vi "XML array.vi"(8 "tag":string, 11 "String":string) -> (3 "Array":string[](array[string]))   [LabVIEW 2013]
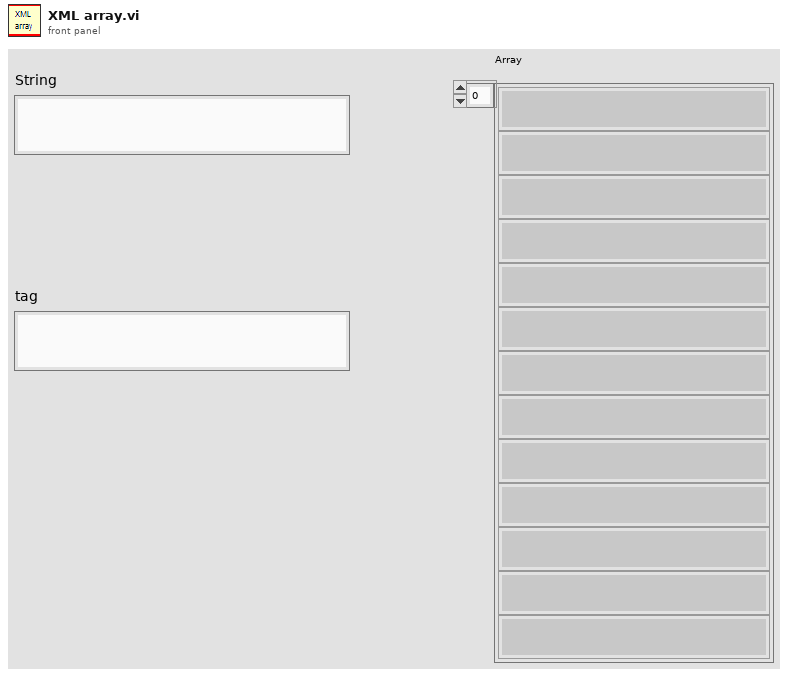
[diagram p1: front panel]
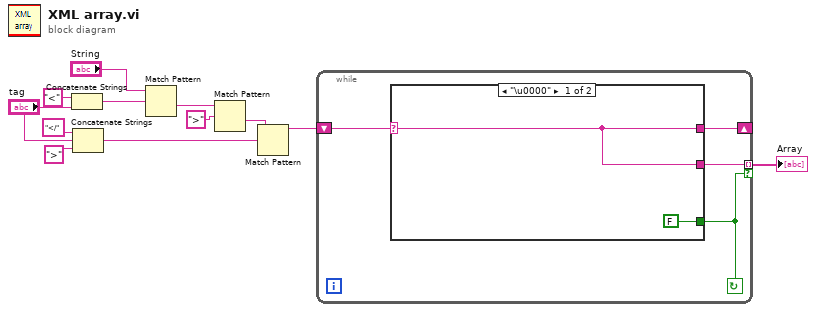
[diagram p0: block diagram]
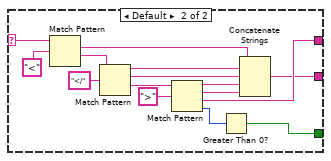
[diagram p2: hidden frame]
diagram:
  n1 = Concatenate Strings("<" ("string"), "tag") -> (w4:string)
  n2 = Concatenate Strings("</" ("string"), "tag", ">" ("string")) -> (w3:string)
  n3 = Match Pattern(string="String", regular expression=w4) -> (after substring=w11:string)  [unwired: 1 in, 3 out]
  n4 = Match Pattern(string=w11, regular expression=">") -> (after substring=w9:string)  [unwired: 1 in, 3 out]
  n5 = Match Pattern(string=w9, regular expression=w3) -> (before substring=w2:string)  [unwired: 1 in, 3 out]
  n6 = while {
    shift-right: [w16] -> _
    shift-left: w2 -> [w14]
    tunnel: [w15] -> w1 mode=indexing if=w13
    stop <- w13 continue-if-true
    n7 = case shown="\"\"" w14 {
      selector: w14 -> [w18 w21]
      tunnel: [w18 w23] -> w16
      tunnel: [w18 w22] -> w15
      tunnel: [FALSE w19] -> w13
      frame "\u0000" {
      }
      frame Default {
        n8 = Match Pattern(string=w21, regular expression="<") -> (match substring=w28:string, after substring=w29:string)  [unwired: 1 in, 2 out]
        n9 = Match Pattern(string=w29, regular expression="</") -> (before substring=w32:string, match substring=w31:string, after substring=w27:string)  [unwired: 1 in, 1 out]
        n10 = Match Pattern(string=w27, regular expression=">") -> (before substring=w25:string, match substring=w24:string, after substring=w23:string, offset past match=w20:i32)  [unwired: 1 in]
        n11 = Greater Than 0?(x=w20) -> (x > 0?=w19:bool)
        n12 = Concatenate Strings(w28, w32, w31, w25, w24) -> (w22:string)
      }
    }
  }
  "Array" <- w1
